vi "BRig_Host__Loop_Producer__tcp_System__Data_storeFiles_buildHeaderLists.vi"(10 "input_arrFilenames":string[](array[string]), 11 "input_nFilenames":i32) -> (2 "output_HeaderLists":string[][](array[string]), 3 "output_HeaderLists":bool[](array[boolean]))   [LabVIEW 2014]
uses:
  <vilib>/Utility/file.llb/Read From Spreadsheet File (string).vi
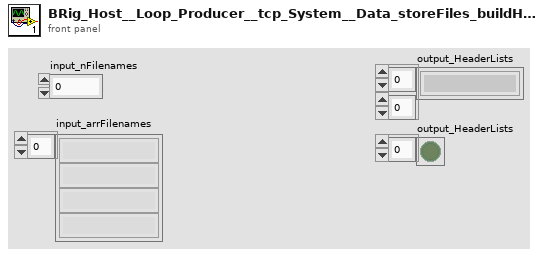
[diagram p1: front panel]
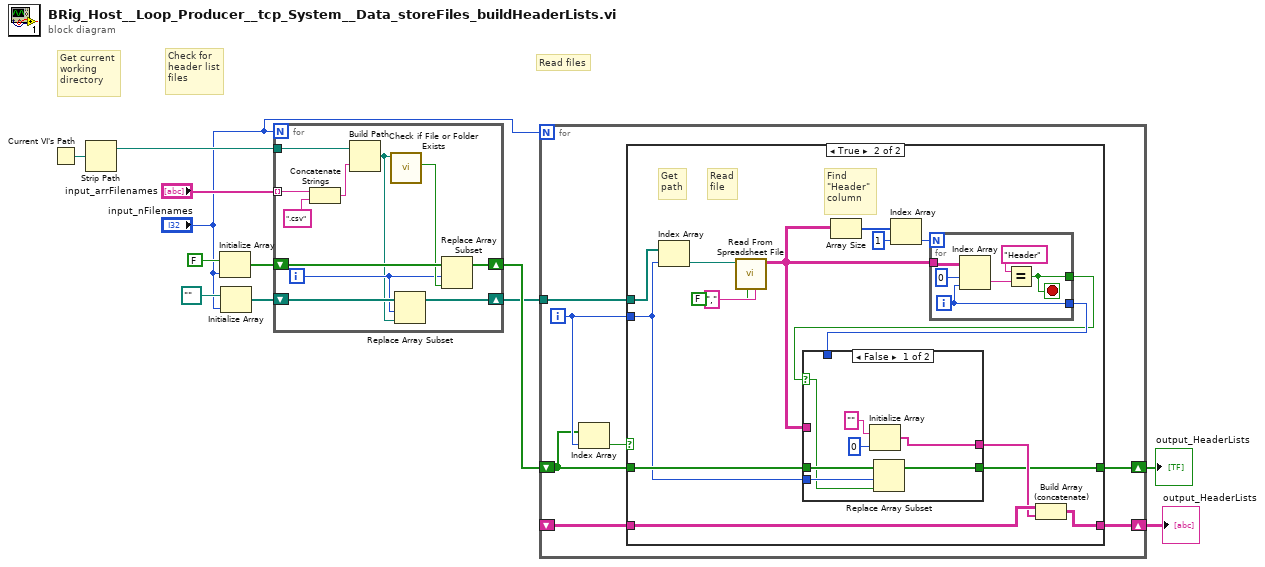
[diagram p0: block diagram]
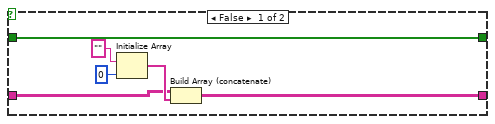
[diagram p2: hidden frame]
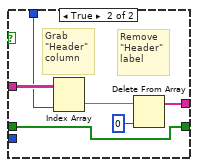
[diagram p3: hidden frame]
diagram:
  # "Read files"
  # "Check for\nheader list\nfiles"
  # "Get current\nworking\ndirectory"
  n1 = Current VI's Path() -> (path=w12:path)
  n2 = Strip Path(path=w12) -> (stripped path=w9:path)  [unwired: 1 out]
  n3 = Initialize Array(FALSE, "input_nFilenames") -> (w8:bool[])
  n4 = Initialize Array(path "" ("path"), "input_nFilenames") -> (w6:path[])
  n5 = for {
    N: "input_nFilenames" -> [_]
    tunnel: "input_arrFilenames" -> [w22] mode=indexing
    tunnel: w9 -> [w23]
    shift-right: [w17] -> w5
    shift-left: w8 -> [w19]
    shift-right: [w15] -> w4
    shift-left: w6 -> [w16]
    i -> [w14]
    n6 = Concatenate Strings(w22, ".csv" ("string")) -> (w20:string)
    n7 = Build Path(base path=w23, name or relative path=w20) -> (appended path=w13:path)
    n8 = call <vilib>:"Check if File or Folder Exists.vi"("path"=w13) -> ("file or folder exists?"=w18:bool)  [unwired: 8 in, 2 out]
    n9 = Replace Array Subset(array=w16, new element=w13, index=w14) -> (w15:path[])
    n10 = Replace Array Subset(array=w19, new element=w18, index=w14) -> (w17:bool[])
  }
  n11 = for {
    N: "input_nFilenames" -> [_]
    tunnel: w4 -> [w30]
    shift-right: [w28] -> w2
    shift-left: _ -> [w29]
    shift-right: [w24] -> w1
    shift-left: w5 -> [w25]
    i -> [w27]
    n12 = Index Array(array=w25, index=w27) -> (element=w26:bool)
    n13 = case shown="True" w26 {
      tunnel: w30 -> [_ w52]
      tunnel: w27 -> [_ w37]
      tunnel: w29 -> [w33 w47]
      tunnel: [w32 w48] -> w28
      tunnel: w25 -> [w31 w39]
      tunnel: [w31 w38] -> w24
      frame False {
        n14 = Initialize Array("", 0 ("dimension size")) -> (w34:string[])
        n15 = Build Array (concatenate)(w33, w34) -> (w32:string[][])
      }
      frame True {
        # "Find\n\"Header\"\ncolumn"
        # "Read\nfile"
        # "Get\npath"
        n16 = Index Array(array=w52, index=w37) -> (element=w51:path)
        n17 = call-poly <vilib>:"Read From Spreadsheet File.vi"("delimiter (\\t)"="," ("delimiter (\\t)"), "transpose (no:F)"=FALSE, "file path (dialog if empty)"=w51) -> ("all rows"=w42:string[][])  [unwired: 4 in, 4 out]
        n18 = Array Size(array=w42) -> (size(s)=w45:i32[])
        n19 = Index Array(array=w45, index=1) -> (element=w43:i32)
        n20 = for {
          N: w43 -> [_]
          tunnel: w42 -> [w71]
          tunnel: [w69] -> w40
          tunnel: [w68] -> w41
          i -> [w68]
          stop <- w69 stop-if-true
          n21 = Index Array(array=w71, index (row)=0 ("disabled index (row)"), index (col)=w68) -> (element=w66:string)
          n22 = Equal?(x="Header" ("y"), y=w66) -> (x = y?=w69:bool)
        }
        n23 = case shown="False" w40 {
          selector: w40 -> [w53 _]
          tunnel: [w57 w63] -> w46
          tunnel: w42 -> [_ w62]
          tunnel: w41 -> [_ w61]
          tunnel: w39 -> [w56 w60]
          tunnel: [w55 w60] -> w38
          tunnel: w37 -> [w54 _]
          frame False {
            n24 = Initialize Array("", 0 ("dimension size")) -> (w57:string[])
            n25 = Replace Array Subset(array=w56, new element=w53, index=w54) -> (w55:bool[])
          }
          frame True {
            # "Remove\n\"Header\"\nlabel"
            # "Grab\n\"Header\"\ncolumn"
            n26 = Index Array(array=w62, index (col)=w61) -> (element=w65:string[])  [unwired: 1 in]
            n27 = Delete From Array(array=w65, index=0) -> (array with subset deleted=w63:string[])  [unwired: 1 in, 1 out]
          }
        }
        n28 = Build Array (concatenate)(w47, w46) -> (w48:string[][])
      }
    }
  }
  "output_HeaderLists" <- w2
  "output_HeaderLists" <- w1
